vi "IO_create_frequency_array.vi"(9 "cor":T1) -> (1 "Array 2":string[](array[string]))   [LabVIEW 2011]
doc: "Creates an array of frequency values corresponding to an input spectrum. Each element in the frequency for each data value in the spectra."
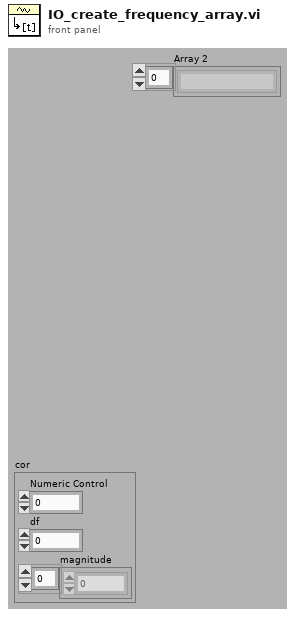
[diagram p1: front panel]
types:
  T1 = cluster{"Numeric Control":dbl, "df":dbl, "magnitude":dbl[]}
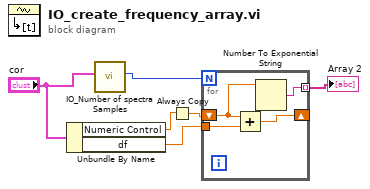
[diagram p0: block diagram]
diagram:
  n1 = Unbundle By Name("cor") -> ("Numeric Control"=w4:dbl, "df"=w5:dbl)
  n2 = call "IO_Number of spectra Samples.vi"("cor"="cor") -> ("number of samples"=w2:i32)  [unwired: 10 in]
  n3 = Always Copy(1:w4) -> (0:w6:dbl)
  n4 = for {
    N: w2 -> [_]
    shift-right: [w9] -> _
    shift-left: w6 -> [w8]
    tunnel: w5 -> [w10]
    tunnel: [w7] -> w1 mode=indexing
    n5 = Add(x=w8, y=w10) -> (x+y=w9:dbl)
    n6 = Number To Exponential String(number=w8) -> (E-format string=w7:string)  [unwired: 3 in]
  }
  "Array 2" <- w1
